vi "Get Names.vi"(10 "Frame Index":u32, 11 "MFStruct Refnum":refnum<vi>) -> (3 "Frame Name":string)   [LabVIEW 2024, in "VI Info.lvlib"]
doc: "This vi determines whether a multi-frame structure is a case structure, event structure, diable structure, or multi-frame sequence, and then gets the name of the frame at the given index using the specific property."
uses:
  <vilib>/Utility/error.llb/Trim Whitespace One-Sided.vi
  VI Info.lvlib
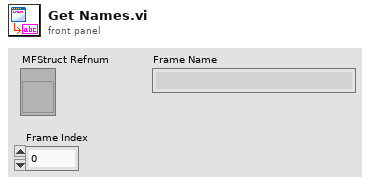
[diagram p1: front panel]
types:
  T1 = enum32{"Conditional Disable Style", "Diagram Disable Style", "Type Specialization Style"}
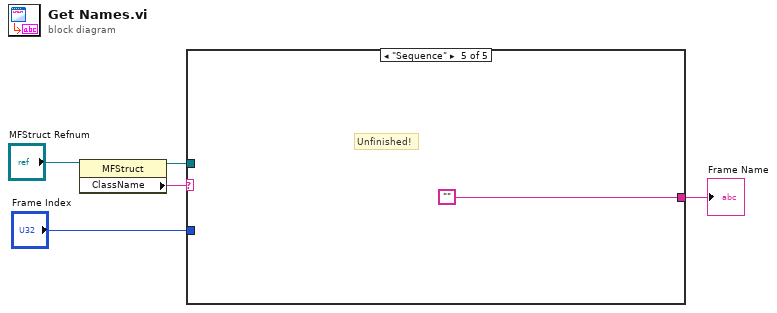
[diagram p0: block diagram]
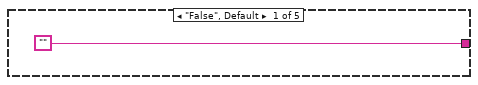
[diagram p2: hidden frame]
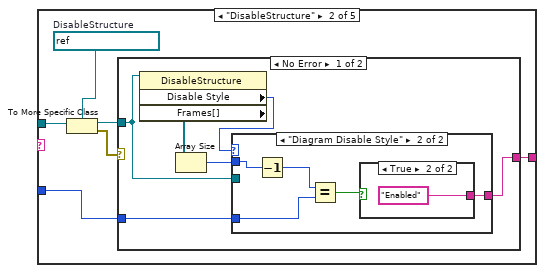
[diagram p3: hidden frame]
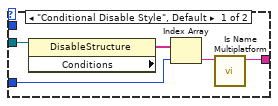
[diagram p4: hidden frame]
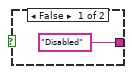
[diagram p5: hidden frame]
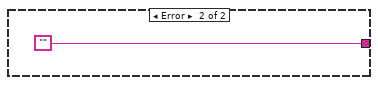
[diagram p6: hidden frame]
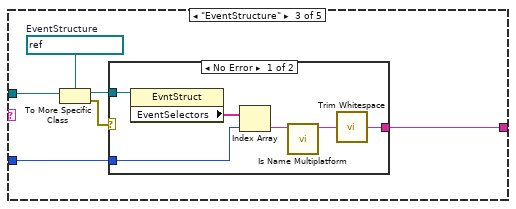
[diagram p7: hidden frame]
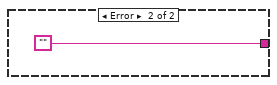
[diagram p8: hidden frame]
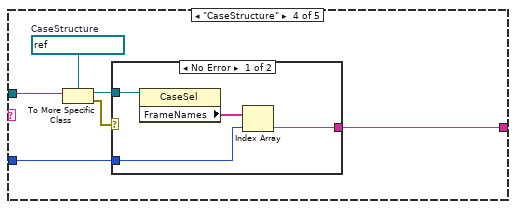
[diagram p9: hidden frame]
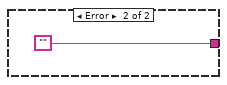
[diagram p10: hidden frame]
diagram:
  n1 = property class="MFStruct"(reference="MFStruct Refnum") -> (reference out=w4:refnum<vi>, "ClassName"=w5:string)  [unwired: 1 in, 1 out]
  n2 = case shown="\"Sequence\"" w5 {
    tunnel: w4 -> [_ w11 w36 w47 _]
    tunnel: ["" w7 w33 w46 ""] -> w1
    tunnel: "Frame Index" -> [_ w8 w32 w45 _]
    frame "False", Default {
    }
    frame "DisableStructure" {
      w12 = refnum<vi> refnum  # DisableStructure
      n3 = To More Specific Class(target class=w12, reference=w11) -> (specific class reference=w10:refnum<vi>, error out=w9:errorcluster)  [unwired: 1 in]
      n4 = case shown="No Error" w9 {
        tunnel: w10 -> [w17 _]
        tunnel: [w18 ""] -> w7
        tunnel: w8 -> [w16 _]
        frame No Error {
          n5 = property class="DisableStructure"(reference=w17) -> ("Disable Style"=w15:T1, "Frames[]"=w14:refnum<vi>[])  [unwired: 1 in, 2 out]
          n6 = Array Size(array=w14) -> (size(s)=w13:i32)
          n7 = case shown="\"Diagram Disable Style\"" w15 {
            tunnel: [w19 w28] -> w18
            tunnel: w17 -> [w22 _]
            tunnel: w16 -> [w20 w26]
            tunnel: w13 -> [_ w27]
            frame "Conditional Disable Style", Default {
              n8 = property class="DisableStructure"(reference=w22) -> ("Conditions"=w21:string[])  [unwired: 1 in, 2 out]
              n9 = Index Array(array=w21, index=w20) -> (element=w23:string)
              n10 = call <vilib>:"Is Name Multiplatform.vi"("filename"=w23) -> ("suggested filename"=w19:string)  [unwired: 6 in, 4 out]
            }
            frame "Diagram Disable Style" {
              n11 = Decrement(x=w27) -> (x-1=w25:i32)
              n12 = Equal?(x=w25, y=w26) -> (x = y?=w24:bool)
              n13 = case shown="True" w24 {
                tunnel: ["Disabled" "Enabled"] -> w28
                frame False {
                }
                frame True {
                }
              }
            }
          }
        }
        frame Error {
        }
      }
    }
    frame "EventStructure" {
      w37 = refnum<vi> refnum  # EventStructure
      n14 = To More Specific Class(target class=w37, reference=w36) -> (specific class reference=w34:refnum<vi>, error out=w35:errorcluster)  [unwired: 1 in]
      n15 = case shown="No Error" w35 {
        tunnel: w34 -> [w41 _]
        tunnel: [w38 ""] -> w33
        tunnel: w32 -> [w40 _]
        frame No Error {
          n16 = property class="EvntStruct"(reference=w41) -> ("EventSelectors"=w43:string[])  [unwired: 1 in, 2 out]
          n17 = Index Array(array=w43, index=w40) -> (element=w42:string)
          n18 = call <vilib>:"Is Name Multiplatform.vi"("filename"=w42) -> ("suggested filename"=w39:string)  [unwired: 6 in, 4 out]
          n19 = call <vilib>:"Trim Whitespace.vi"("string"=w39) -> ("trimmed string"=w38:string)  [unwired: 1 in]
        }
        frame Error {
        }
      }
    }
    frame "CaseStructure" {
      w50 = refnum<vi> refnum  # CaseStructure
      n20 = To More Specific Class(target class=w50, reference=w47) -> (specific class reference=w48:refnum<vi>, error out=w49:errorcluster)  [unwired: 1 in]
      n21 = case shown="No Error" w49 {
        tunnel: w48 -> [w53 _]
        tunnel: [w51 ""] -> w46
        tunnel: w45 -> [w52 _]
        frame No Error {
          n22 = property class="CaseSel"(reference=w53) -> ("FrameNames"=w54:string[])  [unwired: 1 in, 2 out]
          n23 = Index Array(array=w54, index=w52) -> (element=w51:string)
        }
        frame Error {
        }
      }
    }
    frame "Sequence" {
      # "Unfinished!"
    }
  }
  "Frame Name" <- w1
